vi "Initialize.vi"(8 "error in (no error)":errorcluster, 11 "View Template in":refnum<class "[MV] Key Certify.lvclass">) -> (0 "error out":errorcluster, 3 "View Template out":refnum<class "[MV] Key Certify.lvclass">)   [LabVIEW 2020, in "[MV] Key Certify.lvlib" / "[MV] Key Certify.lvclass"]
uses:
  [MV] Key Certify.lvclass
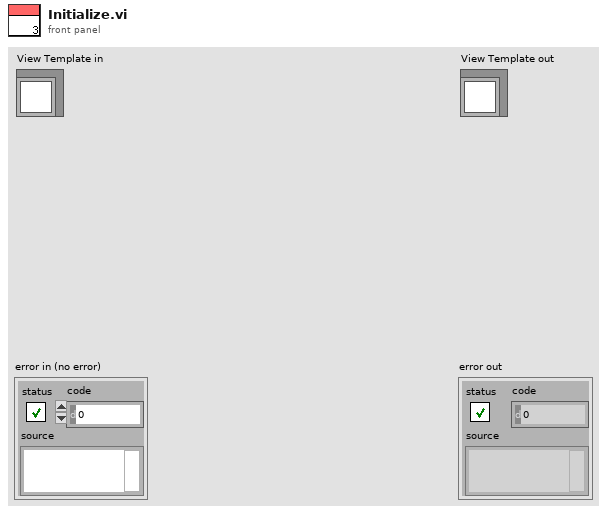
[diagram p1: front panel]
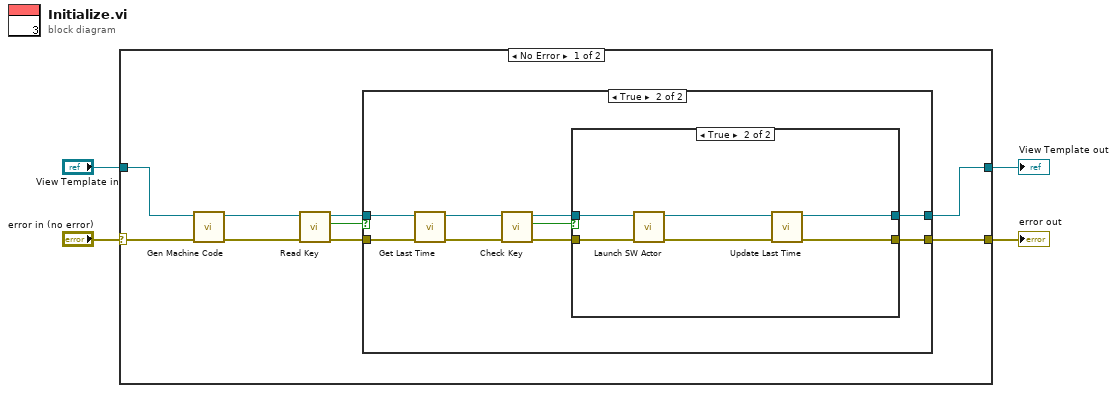
[diagram p0: block diagram]
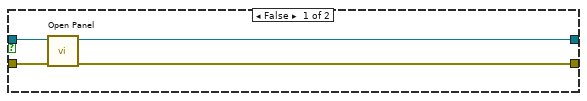
[diagram p2: hidden frame]
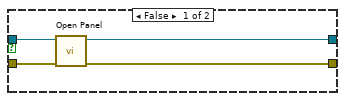
[diagram p3: hidden frame]
diagram:
  n1 = case shown="No Error" "error in (no error)" {
    selector: "error in (no error)" -> [w8 w38]
    tunnel: [w11 w38] -> w3
    tunnel: [w10 w37] -> w1
    tunnel: "View Template in" -> [w5 w37]
    frame No Error {
      n2 = call "Gen Machine Code.vi"("error in (no error)"=w8, "[MV] Key Certify in"=w5) -> ("error out"=w7:errorcluster, "[MV] Key Certify out"=w6:refnum<class "[MV] Key Certify.lvclass">)  [unwired: 8 in]
      n3 = call "Read Key.vi"("error in (no error)"=w7, "[MV] Key Certify in"=w6) -> ("error out"=w12:errorcluster, "exist?"=w13:bool, "[MV] Key Certify out"=w9:refnum<class "[MV] Key Certify.lvclass">)  [unwired: 7 in]
      n4 = case shown="True" w13 {
        tunnel: w12 -> [w17 w24]
        tunnel: w9 -> [w16 w23]
        tunnel: [w15 w25] -> w11
        tunnel: [w14 w26] -> w10
        frame False {
          n5 = call "Open Panel.vi"("error in (no error)"=w17, "[MV] Key Certify in"=w16) -> ("error out"=w15:errorcluster, "[MV] Key Certify out"=w14:refnum<class "[MV] Key Certify.lvclass">)  [unwired: 8 in]
        }
        frame True {
          n6 = call "Get Last Time.vi"("error in (no error)"=w24, "[MV] Key Certify in"=w23) -> ("error out"=w22:errorcluster, "[MV] Key Certify out"=w21:refnum<class "[MV] Key Certify.lvclass">)  [unwired: 8 in]
          n7 = call "Check Key.vi"("error in (no error)"=w22, "[MV] Key Certify in"=w21) -> ("error out"=w20:errorcluster, "valid?"=w18:bool, "[MV] Key Certify out"=w19:refnum<class "[MV] Key Certify.lvclass">)  [unwired: 7 in]
          n8 = case shown="True" w18 {
            tunnel: w20 -> [w30 w36]
            tunnel: w19 -> [w29 w35]
            tunnel: [w28 w31] -> w26
            tunnel: [w27 w32] -> w25
            frame False {
              n9 = call "Open Panel.vi"("error in (no error)"=w30, "[MV] Key Certify in"=w29) -> ("error out"=w27:errorcluster, "[MV] Key Certify out"=w28:refnum<class "[MV] Key Certify.lvclass">)  [unwired: 8 in]
            }
            frame True {
              n10 = call "Launch SW Actor.vi"("error in (no error)"=w36, "[MV] Key Certify in"=w35) -> ("error out"=w34:errorcluster, "[MV] Key Certify out"=w33:refnum<class "[MV] Key Certify.lvclass">)  [unwired: 8 in]
              n11 = call "Update Last Time.vi"("error in (no error)"=w34, "[MV] Key Certify in"=w33) -> ("error out"=w32:errorcluster, "[MV] Key Certify out"=w31:refnum<class "[MV] Key Certify.lvclass">)  [unwired: 8 in]
            }
          }
        }
      }
    }
    frame Error {
    }
  }
  "error out" <- w3
  "View Template out" <- w1
